vi "Get NOK tests from previous DUT.vi"() -> (0 "error IO":errorcluster, 3 "NOK tests from previous DUT":string[](array[string]))   [LabVIEW 2023, in "In a row NOK.lvlib"]
uses:
  In a row NOK.lvlib
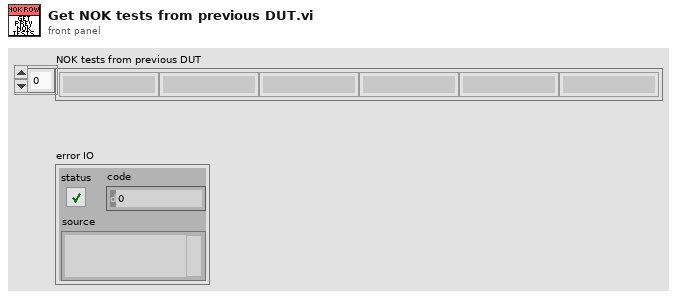
[diagram p1: front panel]
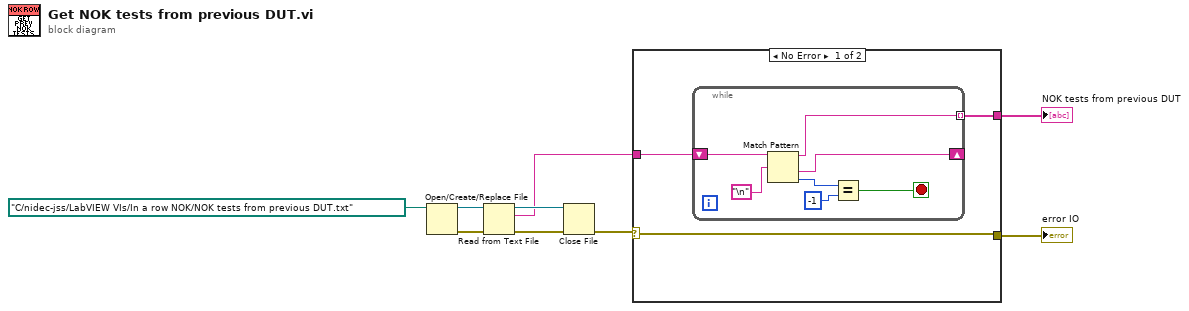
[diagram p0: block diagram]
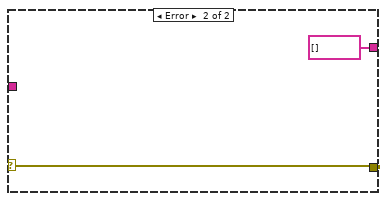
[diagram p2: hidden frame]
diagram:
  n1 = Open/Create/Replace File(file path (use dialog)=path "C:/nidec-jss/LabVIEW VIs/In a row NOK/NOK tests from previous DUT.txt") -> (refnum out=w8:refnum<file>, error out=w7:errorcluster)  [unwired: 5 in, 1 out]
  n2 = Read from Text File(file (use dialog)=w8, error in=w7) -> (refnum out=w6:refnum<file>, text=w4:string, error out=w5:errorcluster)  [unwired: 2 in, 1 out]
  n3 = Close File(refnum=w6, error in=w5) -> (error out=w2:errorcluster)  [unwired: 1 out]
  n4 = case shown="No Error" w2 {
    selector: w2 -> [w10 w21]
    tunnel: w4 -> [w12 _]
    tunnel: [w11 string[] []] -> w3
    tunnel: [w10 w21] -> w1
    frame No Error {
      n5 = while {
        shift-right: [w17] -> _
        shift-left: w12 -> [w19]
        tunnel: [w18] -> w11 mode=indexing
        stop <- w14 stop-if-true
        n6 = Match Pattern(string=w19, regular expression="\n") -> (before substring=w18:string, after substring=w17:string, offset past match=w16:i32)  [unwired: 1 in, 1 out]
        n7 = Equal?(x=w16, y=-1) -> (x = y?=w14:bool)
      }
    }
    frame Error {
    }
  }
  "NOK tests from previous DUT" <- w3
  "error IO" <- w1
